vi "Grab remote image.vi"() -> ()   [LabVIEW 2012]
uses:
  <vilib>/Platform/TimedLoop/XDataNode/timing_clust.ctl
  <vilib>/Platform/TimedLoop/XDataNode/nitl_modes.ctl
  <vilib>/Platform/TimedLoop/XDataNode/wakeup.ctl
  <vilib>/Platform/TimedLoop/XDataNode/XDataNode.xnode
  <vilib>/Platform/TimedLoop/XDataNode/XDNodeRunTimeDep.lvlib
  <vilib>/httpClient/LabVIEWHTTPClient.lvlib
panel:
  out "Vision error":errorcluster
  out "error out 2":errorcluster
  out "HTTP error":errorcluster
  out "headers":string
  out "Image 2":T1(plugin-control)
  out "Image":T1(plugin-control)
  in  "stop":bool
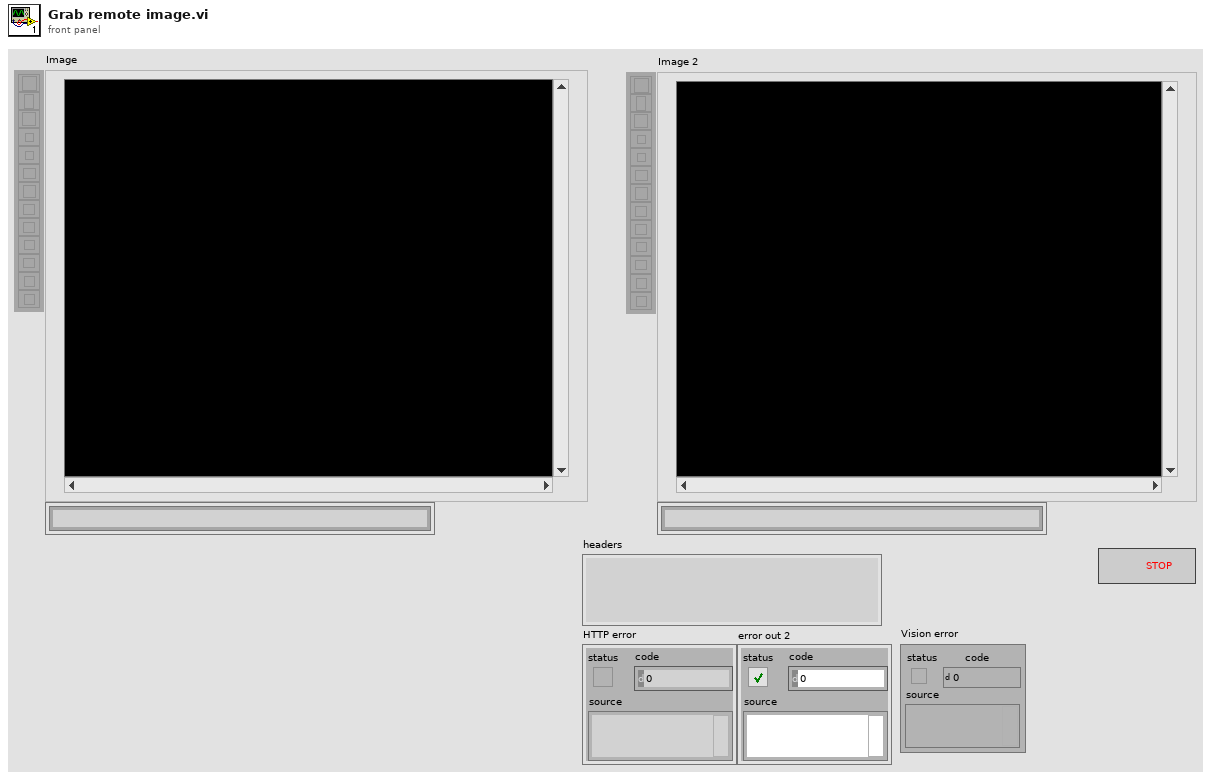
[diagram p1: front panel]
types:
  T1 = typedef "IMAQ Image.ctl" = refnum<image>
  T2 = typedef "XDNodeRunTimeDep.lvlib/timing_clust.ctl" = cluster{"Expected End [f-1]":u64, "Actual End [f-1]":u64, "Finished Late? [f-1]":bool, "Expected End [i-1]":u64, "Actual End [i-1]":u64, "Finished Late? [i-1]":bool, "Expected Start [i]":u64, "Actual Start [i]":u64, "Expected Start [f]":u64, "Actual Start [f]":u64, "Source Name":string, "Structure Name":string, "Period":i64, "Deadline":i64, "Offset":i64, "Start":i64, "Priority":i32, "Timeout":i32, "Mode":T3, "Wakeup Reason":T4, "Error":errorcluster, "Source Type":string, "Secondary Source Type":string, "Global End Time":u64, "Global Start Time":u64, "Frame Duration":u64, "Iteration Duration":u64, "Assigned CPU":i32, "I/O Scan Engine Mode":u32}
  T3 = typedef "XDNodeRunTimeDep.lvlib/nitl_modes.ctl" = enum32{"No Change", "Process missed periods, maintain original phase", "Discard missed periods, maintain original phase", "Process missed periods, ignore original phase", "Discard missed periods, ignore original phase"}
  T4 = typedef "XDNodeRunTimeDep.lvlib/wakeup.ctl" = enum32{"Normal", "Aborted", "Asynchronous wakeup", "Timing source error", "Timed loop error", "Timeout"}
  T5 = typedef "LabVIEWHTTPClient.lvlib/ClientHandle.ctl" = refnum<k1>
  T6 = enum16{"open", "open or create", "create or replace", "create", "open (read only)"}
  T7 = typedef "Image Type" = u32
  T8 = cluster{"Global Rectangle":cluster{"x1Left":i32, "y1Top":i32, "x2Right":i32, "y2Bottom":i32}, "Centroid":cluster{"x":sgl, "y":sgl}, "Object Size":u32, "Score":dbl}[]
  T9 = cluster{"Shape Report (Shape Matching 1)[0]":cluster{"Global Rectangle":cluster{"x1Left":i32, "y1Top":i32, "x2Right":i32, "y2Bottom":i32}, "Centroid":cluster{"x":sgl, "y":sgl}, "Object Size":u32, "Score":dbl}, "Shape Report (Shape Matching 1)[1]":cluster{"Global Rectangle":cluster{"x1Left":i32, "y1Top":i32, "x2Right":i32, "y2Bottom":i32}, "Centroid":cluster{"x":sgl, "y":sgl}, "Object Size":u32, "Score":dbl}, "Shape Report (Shape Matching 1)[2]":cluster{"Global Rectangle":cluster{"x1Left":i32, "y1Top":i32, "x2Right":i32, "y2Bottom":i32}, "Centroid":cluster{"x":sgl, "y":sgl}, "Object Size":u32, "Score":dbl}, "Shape Report (Shape Matching 1)[3]":cluster{"Global Rectangle":cluster{"x1Left":i32, "y1Top":i32, "x2Right":i32, "y2Bottom":i32}, "Centroid":cluster{"x":sgl, "y":sgl}, "Object Size":u32, "Score":dbl}, "Shape Report (Shape Matching 1)[4]":cluster{"Global Rectangle":cluster{"x1Left":i32, "y1Top":i32, "x2Right":i32, "y2Bottom":i32}, "Centroid":cluster{"x":sgl, "y":sgl}, "Object Size":u32, "Score":dbl}, "Shape Report (Shape Matching 1)[5]":cluster{"Global Rectangle":cluster{"x1Left":i32, "y1Top":i32, "x2Right":i32, "y2Bottom":i32}, "Centroid":cluster{"x":sgl, "y":sgl}, "Object Size":u32, "Score":dbl}, "Shape Report (Shape Matching 1)[6]":cluster{"Global Rectangle":cluster{"x1Left":i32, "y1Top":i32, "x2Right":i32, "y2Bottom":i32}, "Centroid":cluster{"x":sgl, "y":sgl}, "Object Size":u32, "Score":dbl}, "Shape Report (Shape Matching 1)[7]":cluster{"Global Rectangle":cluster{"x1Left":i32, "y1Top":i32, "x2Right":i32, "y2Bottom":i32}, "Centroid":cluster{"x":sgl, "y":sgl}, "Object Size":u32, "Score":dbl}, "Shape Report (Shape Matching 1)[8]":cluster{"Global Rectangle":cluster{"x1Left":i32, "y1Top":i32, "x2Right":i32, "y2Bottom":i32}, "Centroid":cluster{"x":sgl, "y":sgl}, "Object Size":u32, "Score":dbl}}
  T10 = cluster{"x1Left":i32, "y1Top":i32, "x2Right":i32, "y2Bottom":i32}
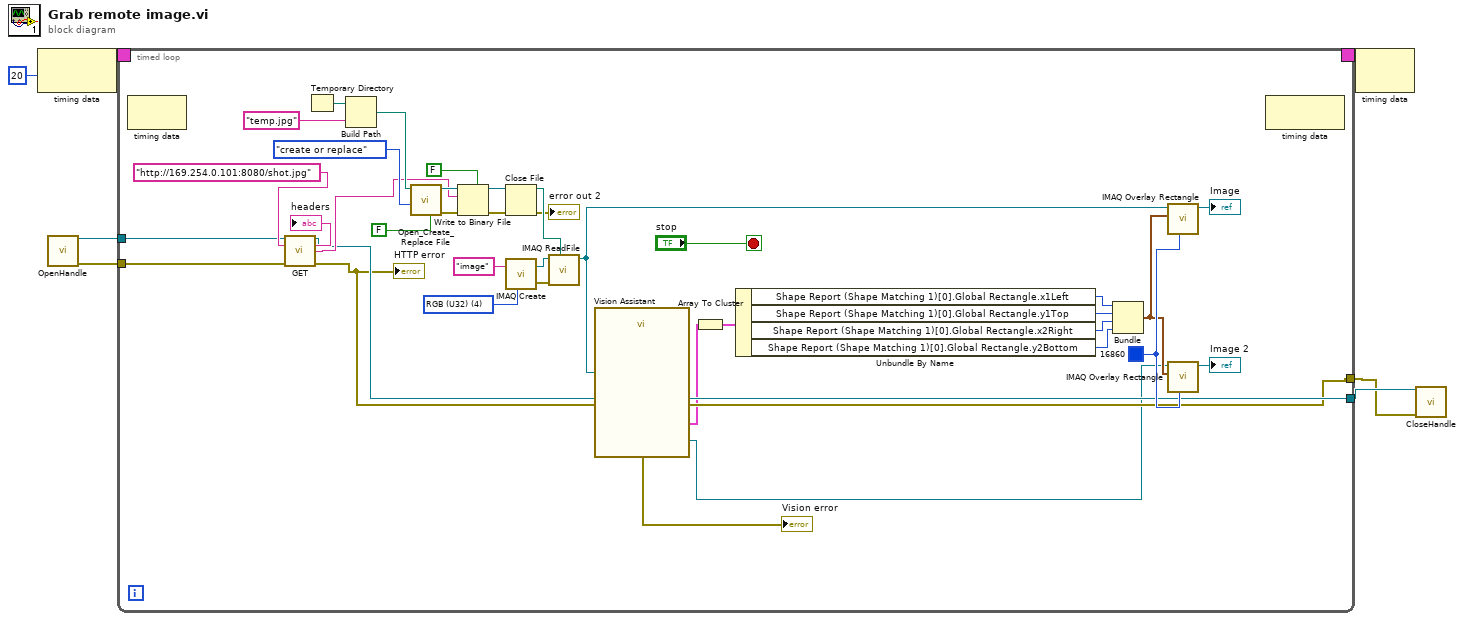
[diagram p0: block diagram]
diagram:
  n1 = node-c288(i64 20 ("Period")) -> (w7:T2)
  n2 = call <vilib>:"OpenHandle.vi"() -> ("client handle out"=w1:T5, "error out"=w2:errorcluster)  [unwired: 14 in]
  n3 = timed-loop {
    timing: w7 -> [_]
    timing-out: [_] -> w6
    tunnel: [w16] -> w4
    tunnel: [w15] -> w3
    tunnel: w2 -> [w9]
    tunnel: w1 -> [w8]
    stop <- "stop" stop-if-true
    w25 = T7 4 items=["Grayscale (U8)", "Grayscale (I16)", "Grayscale (SGL)", "Complex (CSG)", "RGB (U32)", "HSL (U32)", "RGB (U64)", "Grayscale (U16)"] ("Image Type")
    w41 = u32 16860 ("Color")
    n4 = node-c288() -> ()  [unwired: 1 in, 1 out]
    n5 = call <vilib>:"GET.vi"("client handle"=w8, "url"="http://169.254.0.101:8080/shot.jpg", "error in (no error)"=w9) -> ("client handle out"=w16:T5, "headers"=→"headers":string, "body"=w20:string, "error out"=w15:errorcluster)  [unwired: 9 in]
    "HTTP error" <- w15
    n6 = Temporary Directory() -> (w34:path)
    n7 = Build Path(base path=w34, name or relative path="temp.jpg") -> (appended path=w26:path)
    n8 = call <vilib>:"Open_Create_Replace File.vi"("advisory dialog? (display:T)"=FALSE, "function (open:0)"=T6."create or replace", "file path"=w26) -> ("error out"=w31:errorcluster, "refnum"=w32:refnum<file>)  [unwired: 4 in, 3 out]
    n9 = Write to Binary File(file (use dialog)=w32, data=w20, error in=w31, 5:FALSE ("prepend array or string size? (T)")) -> (refnum out=w30:refnum<file>, error out=w29:errorcluster)  [unwired: 3 out]
    n10 = Close File(refnum=w30, error in=w29) -> (path=w22:path, error out=→"error out 2":errorcluster)
    n11 = call "IMAQ Create"("Image Name"="image", "Image Type"=w25) -> ("New Image"=w23:T1, "error out"=w21:errorcluster)  [unwired: 3 in]
    n12 = call "IMAQ ReadFile"("File Path"=w22, "error in (no error)"=w21, "Image"=w23) -> ("Image Out"=w14:T1)  [unwired: 4 in, 4 out]
    n13 = call "Vision Assistant"("Image In"=w14) -> ("Image Out"=w11:T1, "Shape Report (Shape Matching 1)"=w13:T8, "error out"=→"Vision error":errorcluster)  [unwired: 23 in, 1 out]
    n14 = Array To Cluster(array=w13) -> (cluster=w44:T9)
    n15 = Unbundle By Name(w44) -> ("Shape Report (Shape Matching 1)[0].Global Rectangle.x1Left"=w36:i32, "Shape Report (Shape Matching 1)[0].Global Rectangle.y1Top"=w37:i32, "Shape Report (Shape Matching 1)[0].Global Rectangle.x2Right"=w38:i32, "Shape Report (Shape Matching 1)[0].Global Rectangle.y2Bottom"=w39:i32)
    n16 = Bundle("x1Left"=w36, "y1Top"=w37, "x2Right"=w38, "y2Bottom"=w39) -> (w40:T10)  [unwired: 1 in]
    n17 = call "IMAQ Overlay Rectangle"("Color"=w41, "Rectangle"=w40, "Image"=w14) -> ("Image Out"=→"Image":T1)  [unwired: 7 in, 1 out]
    n18 = call "IMAQ Overlay Rectangle"("Color"=w41, "Rectangle"=w40, "Image"=w11) -> ("Image Out"=→"Image 2":T1)  [unwired: 7 in, 1 out]
    n19 = node-c288() -> ()  [unwired: 1 in, 1 out]
  }
  n20 = node-c288(w6) -> ()  [unwired: 1 out]
  n21 = call <vilib>:"CloseHandle.vi"("client handle"=w4, "error in (no error)"=w3) -> ()  [unwired: 13 in, 1 out]
